vi "example_1_nre_vs_re.vi"() -> ()   [LabVIEW 2015, in "lv_mutex_shared_1.lvlib"]
uses:
  lv_mutex_shared_1.lvlib
panel:
  in  "Wait (ms)":u32=1000 min=1
  out "Execution Time (2)":u32
  out "Execution Time (1)":u32
  out "Finish Time (2)":u32
  out "Finish Time (1)":u32
  out "Start Time":u32
  in  "Selection":T1(radio)
  # "This VI will show the difference in execution time for two instances of the\nsame VI running in parallel/simultaneously.  \n\nChange the selection to see the difference.\n*Non ReEntrant execution will take twice as long to execute.\n*ReEntrant execution will take the same amount of time to execute."
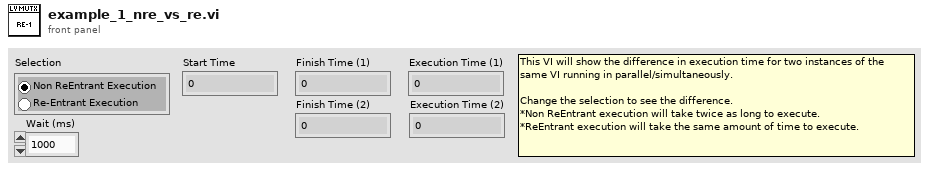
[diagram p1: front panel]
types:
  T1 = enum32{"Non ReEntrant Execution", "Re-Entrant Execution"}
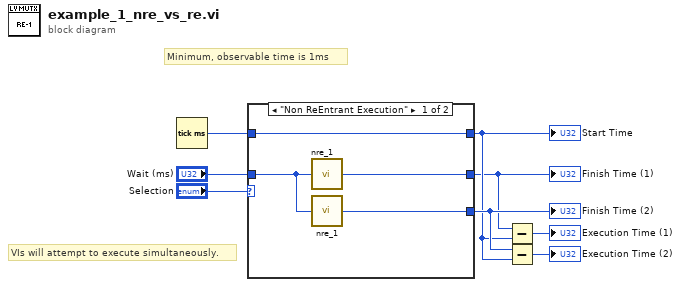
[diagram p0: block diagram]
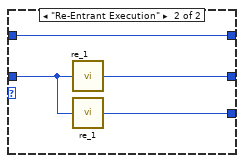
[diagram p2: hidden frame]
diagram:
  # "VIs will attempt to execute simultaneously."
  # "Minimum, observable time is 1ms"
  n1 = Tick Count (ms)() -> (millisecond timer value=w6:u32)
  n2 = case shown="\"Non ReEntrant Execution\"" "Selection" {
    tunnel: "Wait (ms)" -> [w12 w16]
    tunnel: w6 -> [w11 w15]
    tunnel: [w11 w15] -> w2
    tunnel: [w10 w14] -> w1
    tunnel: [w9 w13] -> w3
    frame "Non ReEntrant Execution" {
      n3 = call "nre_1.vi"("wait_ms"=w12) -> ("timer_ms"=w10:u32)
      n4 = call "nre_1.vi"("wait_ms"=w12) -> ("timer_ms"=w9:u32)
    }
    frame "Re-Entrant Execution" {
      n5 = call "re_1.vi"("wait_ms"=w16) -> ("timer_ms"=w14:u32)
      n6 = call "re_1.vi"("wait_ms"=w16) -> ("timer_ms"=w13:u32)
    }
  }
  "Start Time" <- w2
  "Finish Time (1)" <- w1
  "Finish Time (2)" <- w3
  n7 = Subtract(x=w1, y=w2) -> (x-y=→"Execution Time (1)":u32)
  n8 = Subtract(x=w3, y=w2) -> (x-y=→"Execution Time (2)":u32)
